vi "csv_names.vi"(0 "Numeric":i16) -> (1 "concatenated string":string)   [LabVIEW 2015]
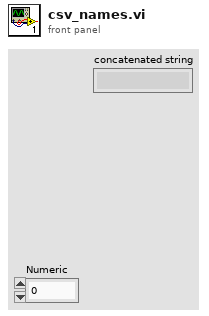
[diagram p1: front panel]
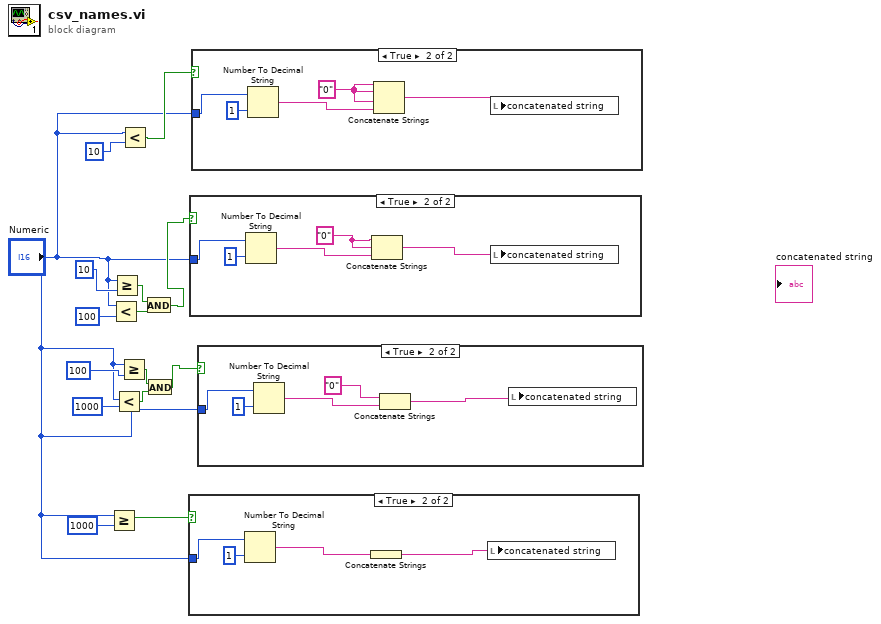
[diagram p0: block diagram]
diagram:
  n1 = Greater Or Equal?(x="Numeric", y=i16 1000) -> (x >= y?=w3:bool)
  n2 = Less?(x="Numeric", y=i16 100) -> (x < y?=w10:bool)
  n3 = Greater Or Equal?(x="Numeric", y=i16 10) -> (x >= y?=w11:bool)
  n4 = Less?(x="Numeric", y=i16 1000) -> (x < y?=w5:bool)
  n5 = Greater Or Equal?(x="Numeric", y=i16 100) -> (x >= y?=w7:bool)
  n6 = Less?(x="Numeric", y=i16 10) -> (x < y?=w12:bool)
  n7 = And(x=w11, y=w10) -> (x .and. y?=w8:bool)
  n8 = And(x=w7, y=w5) -> (x .and. y?=w6:bool)
  n9 = case shown="True" w3 {
    tunnel: "Numeric" -> [_ w16]
    frame False {
    }
    frame True {
      n10 = Number To Decimal String(number=w16, width (-)=i16 1) -> (decimal integer string=w18:string)
      n11 = Concatenate Strings(w18) -> (w17:string)
      n12 = local write "concatenated string"(w17) -> ()
    }
  }
  n13 = case shown="True" w8 {
    tunnel: "Numeric" -> [_ w24]
    frame False {
    }
    frame True {
      w21 = "0" ("string")
      n14 = Number To Decimal String(number=w24, width (-)=i16 1) -> (decimal integer string=w22:string)
      n15 = Concatenate Strings(w21, w21, w22) -> (w20:string)
      n16 = local write "concatenated string"(w20) -> ()
    }
  }
  n17 = case shown="True" w12 {
    tunnel: "Numeric" -> [_ w29]
    frame False {
    }
    frame True {
      w26 = "0" ("string")
      n18 = Number To Decimal String(number=w29, width (-)=i16 1) -> (decimal integer string=w27:string)
      n19 = Concatenate Strings(w26, w26, w26, w27) -> (w25:string)
      n20 = local write "concatenated string"(w25) -> ()
    }
  }
  n21 = case shown="True" w6 {
    tunnel: "Numeric" -> [_ w34]
    frame False {
    }
    frame True {
      n22 = Number To Decimal String(number=w34, width (-)=i16 1) -> (decimal integer string=w32:string)
      n23 = Concatenate Strings("0" ("string"), w32) -> (w30:string)
      n24 = local write "concatenated string"(w30) -> ()
    }
  }
